vi "feature_assemby.vi"(8 "error in (no error)":errorcluster, 11 "Device Out in":T2) -> (0 "error out":errorcluster, 1 "Comm":T3, 2 "value":T1, 3 "Device Out out":T2)   [LabVIEW 2019]
uses:
  <userlib>/IoT Devices/_subVIs/HTTPComm.ctl
  <userlib>/Onshape/_SubVI/Cluster.ctl
  <vilib>/regexp/Match Regular Expression.xnode
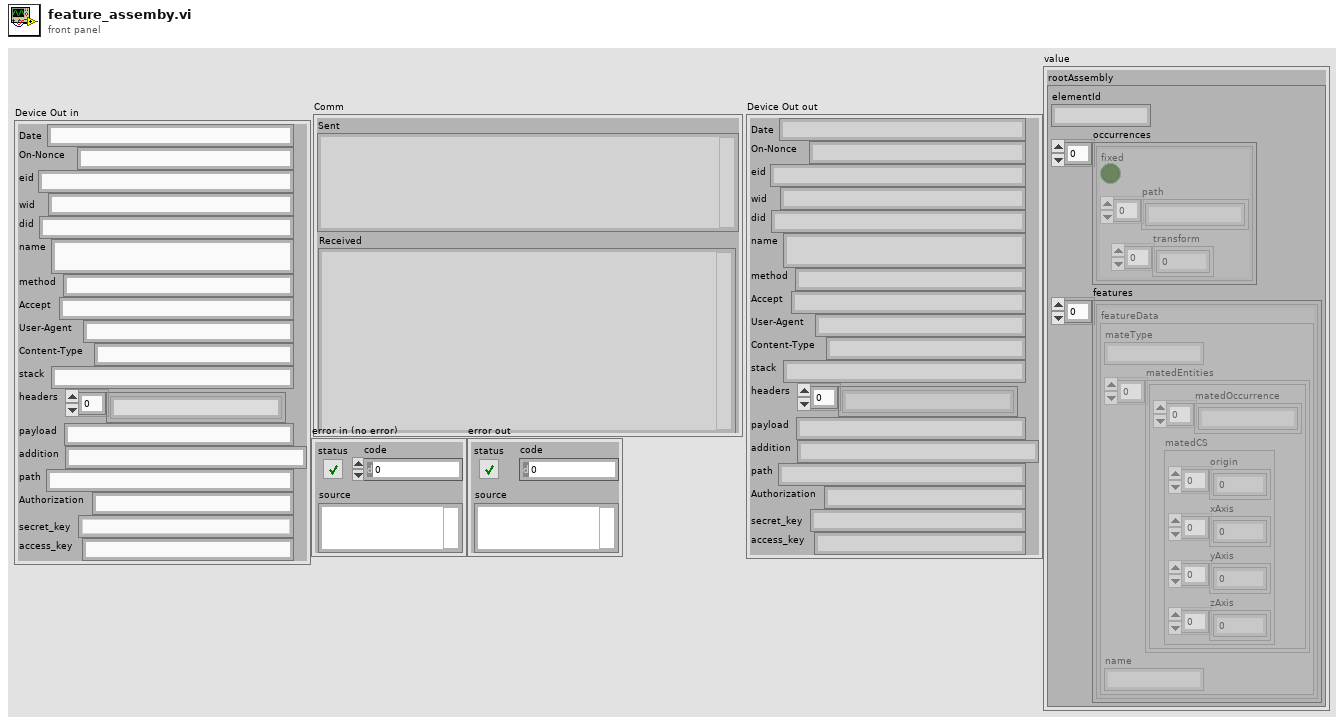
[diagram p1: front panel]
types:
  T1 = cluster{"rootAssembly":cluster{"elementId":string, "occurrences":cluster{"fixed":bool, "path":string[], "transform":dbl[]}[], "features":cluster{"featureData":cluster{"mateType":string, "matedEntities":cluster{"matedOccurrence":string[], "matedCS":cluster{"origin":dbl[], "xAxis":dbl[], "yAxis":dbl[], "zAxis":dbl[]}}[], "name":string}}[]}}
  T2 = typedef "Cluster.ctl" = cluster{"Date":string, "On-Nonce":string, "eid":string, "wid":string, "did":string, "name":string, "method":string, "Accept":string, "User-Agent":string, "Content-Type":string, "stack":string, "headers":string[], "payload":string, "addition":string, "path":string, "Authorization":string, "secret_key":string, "access_key":string}
  T3 = typedef "HTTPComm.ctl" = cluster{"url":string, "sent headers":string, "sent body":string, "headers":string, "body":string, "Sent":string, "Received":string}
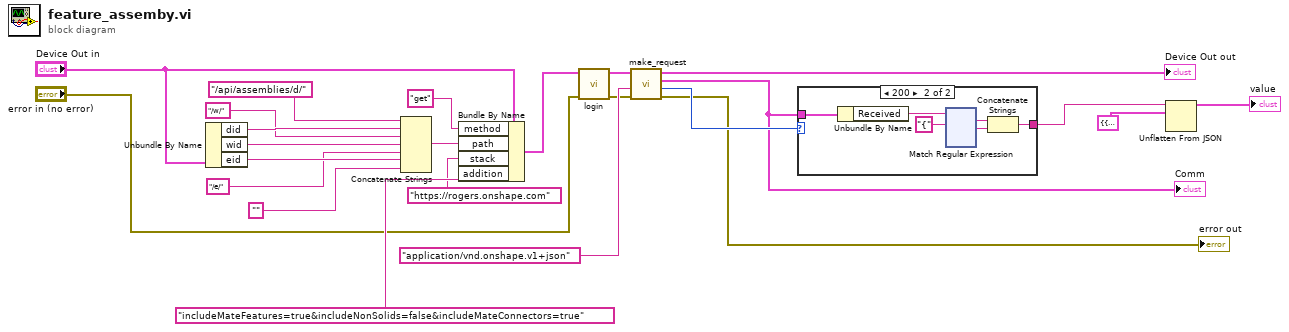
[diagram p0: block diagram]
diagram:
  n1 = Unbundle By Name("Device Out in") -> ("did"=w14:string, "wid"=w15:string, "eid"=w16:string)
  n2 = Concatenate Strings("/api/assemblies/d/" ("payload"), w14, "/w/" ("string"), w15, "/e/" ("string"), w16, "" ("string")) -> (w8:string)
  n3 = Bundle By Name(cluster="Device Out in", "method"="get" ("Method"), "path"=w8, "stack"="https://rogers.onshape.com" ("stacks"), "addition"="includeMateFeatures=true&includeNonSolids=false&includeMateConnectors=true") -> (w17:T2)
  n4 = call <userlib>:"login.vi"("error in"="error in (no error)", "Device In"=w17) -> ("error out"=w12:errorcluster, "Device Out"=w10:T2)  [unwired: 8 in]
  n5 = call <userlib>:"make_request.vi"("Error in"=w12, "Accept"="application/vnd.onshape.v1+json", "Device In"=w10) -> ("error out"=→"error out":errorcluster, "error"=w24:i32, "Comm"=w23:T3, "Device Out"=→"Device Out out":T2)  [unwired: 4 in, 1 out]
  "Comm" <- w23
  n6 = case shown="200" w24 {
    tunnel: w23 -> [_ w30]
    tunnel: [_ w25] -> w3
    frame 0, Default {
    }
    frame 200 {
      n7 = Unbundle By Name(w30) -> ("Received"=w26:string)
      n8 = xnode "Match Regular Expression"("input string"=w26, "regular expression"="{" ("search string")) -> ("whole match"=w28:string, "after match"=w27:string)  [unwired: 4 in, 3 out]
      n9 = Concatenate Strings(w28, w27) -> (w25:string)
    }
  }
  n10 = Unflatten From JSON(JSON string=w3, type and defaults=T1 {"rootAssembly"={"elementId"="", "occurrences"=[], "features"=[]}}) -> (value=→"value":T1)  [unwired: 5 in, 1 out]
